vi "Micro-PL v10.4.1.vi"() -> ()   [LabVIEW 2010]
uses:
  drivers/Oxford ITC/ITCAPPS.LLB/ITCSetup.ctl
  drivers/Oxford ITC/ITCSUBS.LLB/ITCIO.ctl
  drivers/Oxford ITC/BUSGEN.LLB/OxfordAddress.ctl
  drivers/Oxford ITC/ITCSUBS.LLB/ITCVersion.ctl
  subvi/ESA-C/TypeDefs/ESA-C Live Controls v10.4.0.ctl
  subvi/ESA-C/TypeDefs/ESA-C Current Values.ctl
  subvi/ESA-C/TypeDefs/ESA-C Connection Settings.ctl
  subvi/ESA-C/TypeDefs/ESA-C Set Positions.ctl
  subvi/ITC503/TypeDefs/ITC503 Settings.ctl
  subvi/ITC503/TypeDefs/ITC503 Current Values.ctl
  subvi/iHR550/TypeDefs/iHR Current Values.ctl
  subvi/iHR550/TypeDefs/iHR Settings.ctl
  subvi/Mapping/TypeDefs/Mapping Spectra Params.ctl
  <vilib>/Utility/miscctls.llb/LVBoundsTypeDef.ctl
  <vilib>/Utility/miscctls.llb/LVPointTypeDef.ctl
  drivers/Horiba Spectrum One 3000V/Lib/CCD_command.llb/Comm Params.ctl
  subvi/Global Variables.vi
  <vilib>/Analysis/NI_AALBase.lvlib
panel:
  out "Spectrum Raw":dbl[][](array[numeric])
  out "Mapping State Storage":bool
  out "Mapping Reference":refnum<vi>
  out "Copy Drive Target":bool
  in  "CCD3500 Shutter":bool caption="Shutter:"
  out "Measurement Running":bool
  out "ITC503s Running":bool
  out "Drive Running":bool
  out "CCD3500V Running":bool
  out "iHR550 Running":bool
  in  "Exit":bool
  out "iHR550 Status":bool
  out "Drive Status":bool
  out "CCD3500V Status":bool
  out "ITC503 Status":bool
  in  "Register":enum32{"Devices", "Acquisition / Mapping"}(tab)
  out "iHR550 Timing":u32 caption="iHR550"
  out "Drive Timing":u32 caption="Drive"
  out "ITC Timing":u32 caption="ITC"
  out "CCD Timing":u32 caption="CCD"
  out "CCD3500 Temperature":dbl caption="Temp. (°C)" min=10.0 max=160.0 step=0.1 format="%.1f"
  in  "CCD3500V GPIB-Port":i32=5 caption="GPIB-Port" min=1 max=20 step=1 format="%#.0f"
  in  "CCD3500V Connect":bool
  in  "iHR550 Force Init":bool=TRUE
  in  "iHR550 Connect":bool
  in  "iHR550 ID":string(combo)="iHR550" caption="Monochromator ID"
  out "ITC503 Current Values":T1 {"ITC503 Gradient" format="%.2f"; "ITC503 Setpoint" min=-273.0 max=300000.0 step=0.0001 format="%.1f"; "ITC503 I" format="%_1f"; "ITC503 P" format="%_1f"; "ITC503 Temperature" min=0.0 max=1645.0 step=1e-05 format="%.2f"; "ITC503 Heater" min=0.0 max=100.0 step=0.01 scale=0.0..100.0}
  in  "ITC503 Settings":T2={"ITC503 Set Setpoint"=0.0, "ITC503 Set Auto Heater"=TRUE, "ITC503 Set Auto PID"=TRUE, "P"=0.0, "I"=0.0, "D"=0.0} {"D" min=0.0 max=100.0 step=0.1 format="%.1f"; "I" min=0.0 max=100.0 step=0.1 format="%.1f"; "P" min=0.0 max=100.0 step=0.1 format="%.1f"; "ITC503 Set Setpoint" min=-273.0 max=300000.0 step=0.1 format="%.1f"}
  in  "ITC503 Configure":bool
  in  "ITC503 Connect":bool
  in  "ITC503 Selector":u16(ring) caption="Select Device" items=["ITC503s"]
  out "Drive Current Values":T3 {"Position"."Drive Z Position" min=-273.0 max=300000.0 step=0.0001 format="%.1f"; "Position"."Drive Y Position" min=-273.0 max=300000.0 step=0.0001 format="%.1f"; "Position"."Drive X Position" min=-273.0 max=300000.0 step=0.0001 format="%.1f"; "Voltages"."Drive Z Voltage" min=-273.0 max=300000.0 step=0.0001 format="%.1f"; "Voltages"."Drive Y Voltage" min=-273.0 max=300000.0 step=0.0001 format="%.1f"; "Voltages"."Drive X Voltage" min=-273.0 max=300000.0 step=0.0001 format="%.1f"}
  in  "Drive Connection":T4={"Objective GPIB-Port"=4, "Stage GPIB-Port"=4, "Drive Selector"=0, "Drive Velocity (V/s)"=5.0} {"Drive Velocity (V/s)" min=10.0 max=160.0 step=0.1 format="%.1f"; "Drive Selector" items=["Obj.", "Stage"]; "Stage GPIB-Port" min=1 max=20 step=1 format="%#.0f"; "Objective GPIB-Port" min=1 max=20 step=1 format="%#.0f"}
  in  "Drive Connect":bool
  in  "Snapshot Folder":path=path "C:/Users/WET-KORR/Desktop/Screenshots"
  in  "Camera Name":string="HD USB Camera"
  in  "Spectrum Noise":i64 caption="Noise Level"
  in  "Wavelength Switch":bool
  out "Spectrum":cluster{dbl[], dbl[]}[](graph)
  in  "Spectrum Load":bool
  in  "Spectrum Save":bool
  in  "CCD3000 Current Rep.":string="0/0"
  in  "Spectrum Maximize":bool
  in  "Video Show":bool
  in  "Drive GoTo":bool caption="Objective Move Abs."
  in  "Drive New Positions":T5 {"Drive X Set" min=10.0 max=160.0 step=0.1 format="%.1f"; "Drive Z Set" min=10.0 max=160.0 step=0.1 format="%.1f"; "Drive Y Set" min=10.0 max=160.0 step=0.1 format="%.1f"}
  in  "Spectrum Autosave":bool caption="iHR550 Force Init"
  in  "CCD3500 Preview":bool
  in  "CCD3500 Acquire":bool
  in  "Spectra Settings":T6={"Integration Time"=1.0, "Repetitions"=1, "Mapping Spectra"=TRUE} caption="Mapping Spectra Settings" {"Repetitions" min=1 max=100 step=1; "Integration Time" min=0.1 max=6000.0 step=0.1 format="%.1f"}
  in  "Mapping Start":bool
  in  "iHR550 Configure":bool
  in  "iHR Settings":T7={"iHR550 Set Exit Mirror"=2, "iHR550 Set Side Exit"=0.0, "iHR550 Set Front Entrance"=0.0, "iHR550 Set Wavelength"=897.9988, "iHR550 Set Grating"=0, "iHR550 Set Grating Switch"=FALSE, "iHR550 Set Wavelength Switch"=FALSE, "iHR550 Set Mirror Switch"=FALSE, "iHR550 Set Slits Switch"=FALSE} {"iHR550 Set Grating" items=["1800"=1, "600"=2, "150"=3]; "iHR550 Set Wavelength" min=0.0 max=1500.0 step=1.0; "iHR550 Set Side Exit" min=0.0 max=2000.0 step=1.0; "iHR550 Set Exit Mirror" items=["Front"=2, "Side"=3]}
  out "iHR Current Values":T8={"iHR 550 Front Entrance"=0.0, "iHR550 Side Exit"=0.0, "iHR550 Wavelength"=897.9988, "iHR550 Exit Mirror"=2, "iHR550 Grating"="1", "Grating Index"=1} {"iHR550 Exit Mirror" items=["EntranceMirror", "ExitMirror", "Front", "Side"]}
  out "Drive Live Current Values":T3 {"Position"."Drive Z Position" min=-273.0 max=300000.0 step=0.0001 format="%.1f"; "Position"."Drive Y Position" min=-273.0 max=300000.0 step=0.0001 format="%.1f"; "Position"."Drive X Position" min=-273.0 max=300000.0 step=0.0001 format="%.1f"; "Voltages"."Drive Z Voltage" min=-273.0 max=300000.0 step=0.0001 format="%.1f"; "Voltages"."Drive Y Voltage" min=-273.0 max=300000.0 step=0.0001 format="%.1f"; "Voltages"."Drive X Voltage" min=-273.0 max=300000.0 step=0.0001 format="%.1f"}
  in  "Drive Live Controls":T9={"Move Step"=1.0, "Move Home"=FALSE, "Move Down"=FALSE, "Move Up"=FALSE, "Move Left"=FALSE, "Move Right"=FALSE, "Move Out"=FALSE, "Move In"=FALSE} {"Move Step" min=0.0 max=30.0 step=0.1 format="%.1f"}
  out "ITC503 Temp Storage":dbl
  out "Runtime":u32
  out "ITC Gradient Time":i64
  out "Read ITC":bool
  out "Read CCD3500":bool
  out "Read iHR550":bool
  out "Read Drive":bool
  out "Spectrum Properties":cluster{"Position":T10, "Plot Area Size":T10}={"Position"={"Width"=36, "Height"=367}, "Plot Area Size"={"Width"=496, "Height"=264}}
  in  "Auto Folder":path caption="Ausgewählter Pfad"
  out "Int. Time Temp":dbl
  out "Wavelengths (nm)":dbl[](array[numeric])
  in  "CCD3500V Connection":T11={"Comm Interface"=1, "BUS"=0, "Address"=5, "Com Port"=0}
  out "Video Running":bool
  out "iHR550 RefNum":refnum<k7> caption="Mono RefNum out"
  out "ITC Setup":T12={"Description"="", "IO Info"={"Address"={"Com Port"=1, "ISOBUS Address"=1, "GPIB Address"=24, "Communication"=enum."ISOBUS"}, "Version"=enum."ITC503", "Ch 1 dec places"=1, "Ch 2 dec places"=1, "Ch 3 dec places"=1, "Ch1 Name"="", "Ch2 Name"="", "Ch3 Name"=""}}
  # "Correlation Setup"
  # "Active"
  # "Active"
  # "ITC"
  # "iHR"
  # "Drive"
  # "CCD"
  # "Status"
  # "CCD"
  # "ITC"
  # "iHR"
  # "Drive"
  # "Timing"
  # "CCD"
  # "Monochromator"
  # "Cryostat"
  # "Drives"
  # "Video"
  # "Drive Control"
  # "Spectrum"
  # "CCD"
  # "Mapping"
  # "Launch the Spectral Mapping VI and Raman Tool Set 2.0 in a new window."
  # "Monochromator"
  # "XY"
  # "Z"
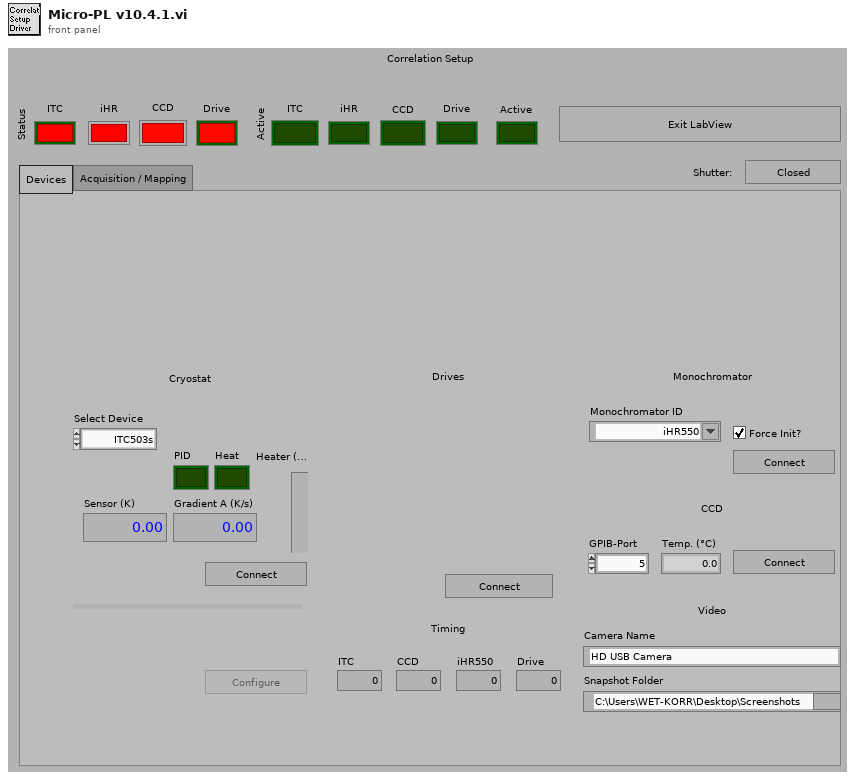
[diagram p1: front panel]
types:
  T1 = typedef "ITC503 Current Values.ctl" = cluster{"ITC503 Heater":dbl, "ITC503 Temperature":dbl, "ITC503 P":dbl, "ITC503 I":dbl, "ITC503 D":dbl, "ITC503 Setpoint":dbl, "ITC503 Gradient":dbl, "ITC503 Heater Auto":bool, "ITC503 PID Auto":bool}
  T2 = typedef "ITC503 Settings.ctl" = cluster{"ITC503 Set Setpoint":dbl, "ITC503 Set Auto Heater":bool, "ITC503 Set Auto PID":bool, "P":dbl, "I":dbl, "D":dbl}
  T3 = typedef "ESA-C Current Values.ctl" = cluster{"Voltages":cluster{"Drive X Voltage":dbl, "Drive Y Voltage":dbl, "Drive Z Voltage":dbl}, "Position":cluster{"Drive X Position":dbl, "Drive Y Position":dbl, "Drive Z Position":dbl}}
  T4 = typedef "ESA-C Connection Settings.ctl" = cluster{"Objective GPIB-Port":i32, "Stage GPIB-Port":i32, "Drive Selector":u16, "Drive Velocity (V/s)":dbl}
  T5 = typedef "ESA-C Set Positions.ctl" = cluster{"Drive X Set":dbl, "Drive Y Set":dbl, "Drive Z Set":dbl}
  T6 = typedef "Mapping Spectra Params.ctl" = cluster{"Integration Time":dbl, "Repetitions":u16, "Mapping Spectra":bool}
  T7 = typedef "iHR Settings.ctl" = cluster{"iHR550 Set Exit Mirror":u16, "iHR550 Set Side Exit":dbl, "iHR550 Set Front Entrance":dbl, "iHR550 Set Wavelength":dbl, "iHR550 Set Grating":u16, "iHR550 Set Grating Switch":bool, "iHR550 Set Wavelength Switch":bool, "iHR550 Set Mirror Switch":bool, "iHR550 Set Slits Switch":bool}
  T8 = typedef "iHR Current Values.ctl" = cluster{"iHR 550 Front Entrance":dbl, "iHR550 Side Exit":dbl, "iHR550 Wavelength":dbl, "iHR550 Exit Mirror":i32, "iHR550 Grating":string, "Grating Index":i32}
  T9 = typedef "ESA-C Live Controls v10.4.0.ctl" = cluster{"Move Step":dbl, "Move Home":bool, "Move Down":bool, "Move Up":bool, "Move Left":bool, "Move Right":bool, "Move Out":bool, "Move In":bool}
  T10 = typedef "LVBoundsTypeDef.ctl" = cluster{"Width":u32, "Height":u32}
  T11 = cluster{"Comm Interface":u16, "BUS":i16, "Address":i16, "Com Port":i32}
  T12 = typedef "ITCSetup.ctl" = cluster{"Description":string, "IO Info":T13}
  T13 = typedef "ITCIO.ctl" = cluster{"Address":T14, "Version":T15, "Ch 1 dec places":i16, "Ch 2 dec places":i16, "Ch 3 dec places":i16, "Ch1 Name":string, "Ch2 Name":string, "Ch3 Name":string}
  T14 = typedef "OxfordAddress.ctl" = cluster{"Com Port":i32, "ISOBUS Address":i32, "GPIB Address":i16, "Communication":enum16{"RS232", "ISOBUS", "GPIB", "Gateway"}}
  T15 = typedef "ITCVersion.ctl" = enum16{"ITC502", "ITC503", "ITC601"}
  T16 = typedef "LVPointTypeDef.ctl" = cluster{"Horizontal":i16, "Vertical":i16}
  T17 = enum8{"Enabled", "Disabled", "Disabled and Grayed Out"}
  T18 = typedef "Comm Params.ctl" = cluster{"Comm Interface":u16, "BUS":i16, "Address":i16, "Com Port":i32}
  T19 = enum16{"CCD Temperature Z345", "CCD Temperature Z308", "CCD Gain"}
  T20 = cluster{"CCD3000 Connection":T18, "Drive Connection Settings":T4, "ITC503 Current Values":T1, "Wavelengths (nm)":dbl[], "Drive Current Values":T3, "iHR Current Values":T8, "Spectra Settings":T6, "CCD3500 Temperature":dbl, "Simulate Drive 2":bool, "Simulate Spectra 2":bool}
  T21 = cluster{"Drive X Position":dbl, "Drive Y Position":dbl, "Drive Z Position":dbl}
  T22 = cluster{"Intensities":dbl[], "Wavelengths":dbl[]}[]
  T23 = typedef "LVPositionTypeDef.ctl" = cluster{"Left":i32, "Top":i32}
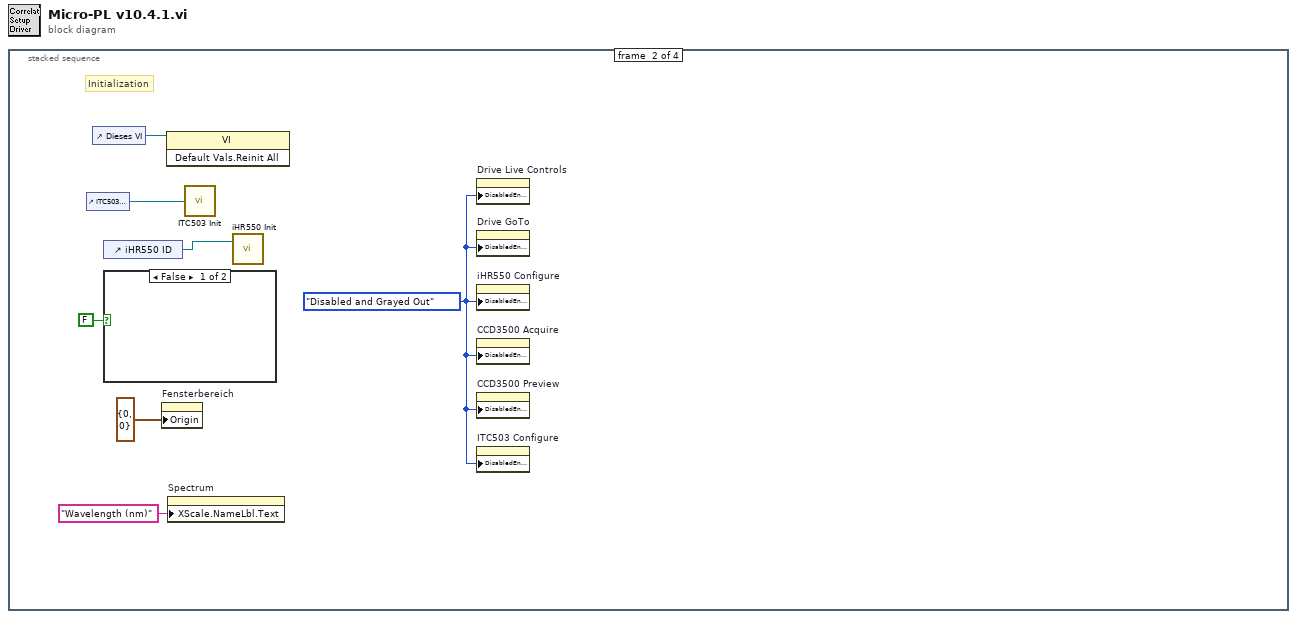
[diagram p0: block diagram]
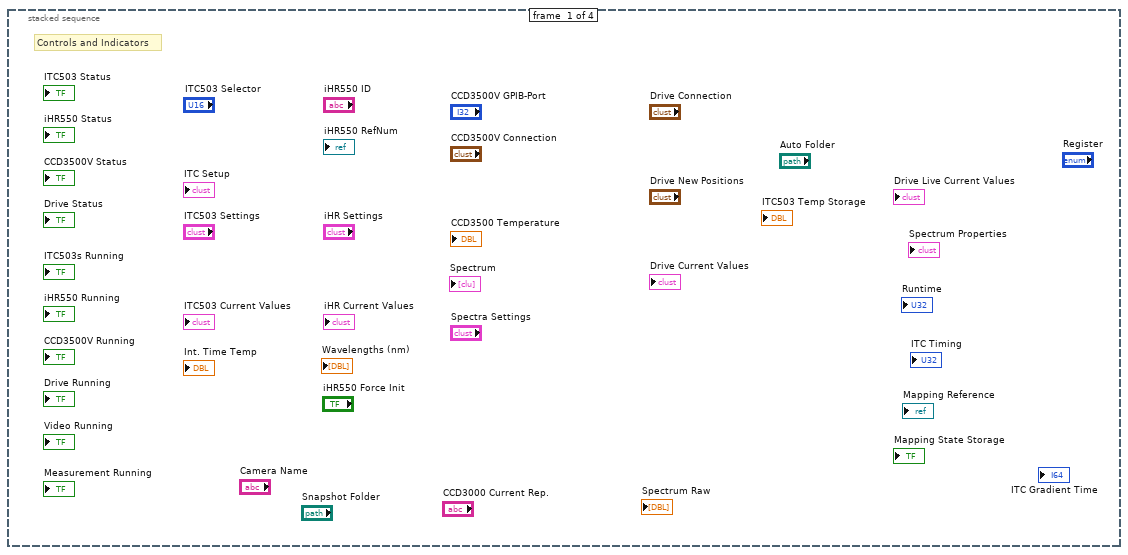
[diagram p2: hidden frame]
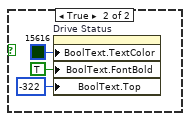
[diagram p3: hidden frame]
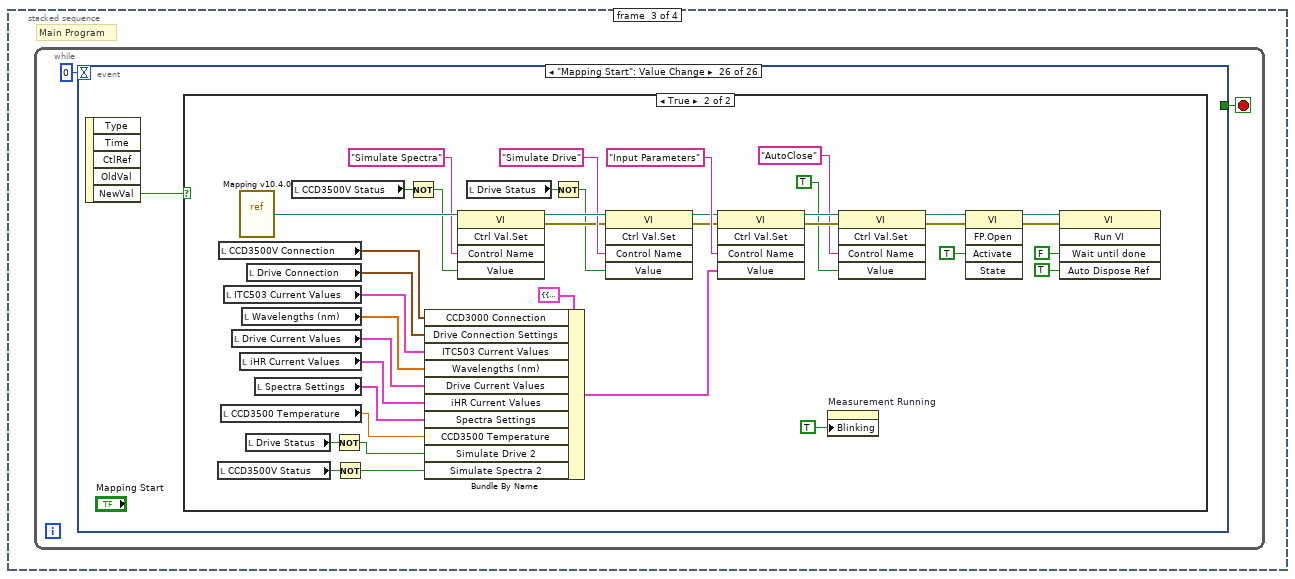
[diagram p4: hidden frame]
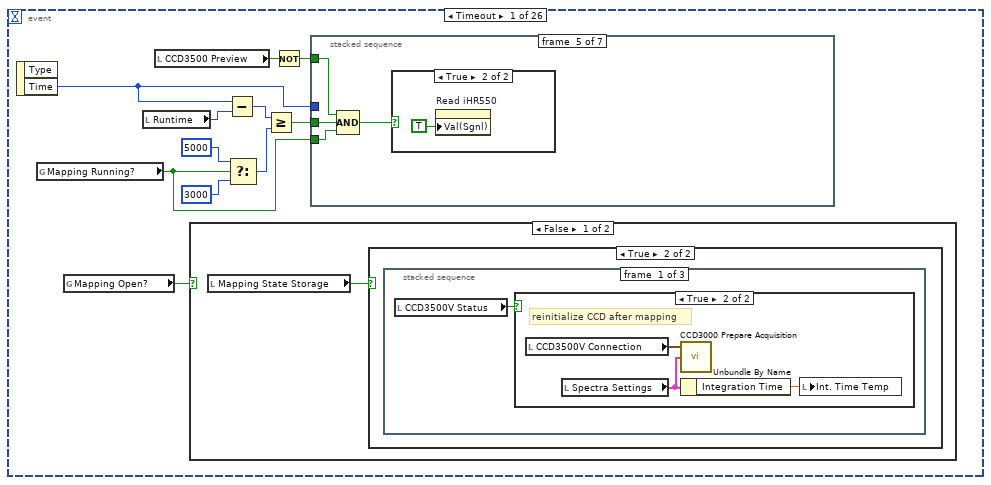
[diagram p5: hidden frame]
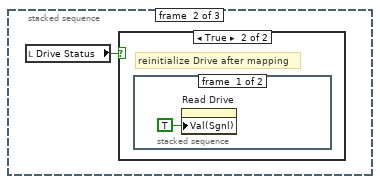
[diagram p8: hidden frame]
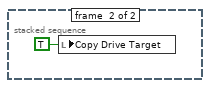
[diagram p10: hidden frame]
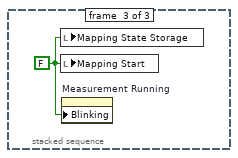
[diagram p11: hidden frame]
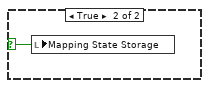
[diagram p12: hidden frame]
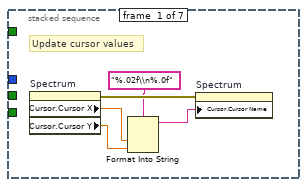
[diagram p13: hidden frame]
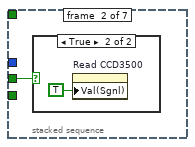
[diagram p14: hidden frame]
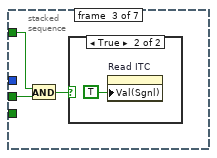
[diagram p16: hidden frame]
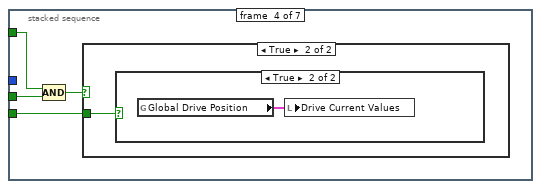
[diagram p18: hidden frame]
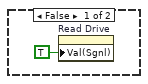
[diagram p20: hidden frame]
diagram:
  n1 = stacked-sequence {
    frame #0 {
      # "Controls and Indicators"
    }
    frame #1 {
      w2 = T17."Disabled and Grayed Out" ("Deaktiviert")
      # "Initialization"
      n2 = control-ref of="ITC503 Selector"() -> (w7:refnum<vi>)
      n3 = control-ref of="Dieses VI"() -> (w6:refnum<vi>)
      n4 = control-ref of="iHR550 ID"() -> (w5:refnum<vi>)
      n5 = case shown="False" FALSE {
        frame False {
        }
        frame True {
          n6 = property on="Drive Status" class="Bool (strict)"("BoolText.TextColor"=u32 15616, "BoolText.FontBold"=TRUE ("Boolescher Text.Schriftart:Fett"), "BoolText.Top"=-322 ("Boolescher Text.Position:Oben")) -> ()  [unwired: 2 in, 2 out]
        }
      }
      n7 = property on="Fensterbereich" class="Pane"("Origin"=T16 {"Horizontal"=0, "Vertical"=0}) -> ()  [unwired: 2 in, 2 out]
      n8 = invoke class="VI" method="Default Vals.Reinit All"(reference=w6) -> ()  [unwired: 2 in, 3 out]
      n9 = property on="Spectrum" class="XYGraph (strict)"("XScale.NameLbl.Text"="Wavelength (nm)" ("X Scale.Name Label.Text")) -> ()  [unwired: 2 in, 2 out]
      n10 = call "ITC503 Init.vi"("ITC Selector"=w7) -> ()  [unwired: 1 in]
      n11 = call "iHR550 Init.vi"("Mono ID"=w5) -> ()  [unwired: 2 in]
      n12 = property on="Drive Live Controls" class="Clust (strict)"("DisabledEnum"=w2) -> ()  [unwired: 2 in, 2 out]
      n13 = property on="Drive GoTo" class="Bool (strict)"("DisabledEnum"=w2) -> ()  [unwired: 2 in, 2 out]
      n14 = property on="iHR550 Configure" class="Bool (strict)"("DisabledEnum"=w2) -> ()  [unwired: 2 in, 2 out]
      n15 = property on="CCD3500 Acquire" class="Bool (strict)"("DisabledEnum"=w2) -> ()  [unwired: 2 in, 2 out]
      n16 = property on="CCD3500 Preview" class="Bool (strict)"("DisabledEnum"=w2) -> ()  [unwired: 2 in, 2 out]
      n17 = property on="ITC503 Configure" class="Bool (strict)"("DisabledEnum"=w2) -> ()  [unwired: 2 in, 2 out]
    }
    frame #2 {
      # "Main Program"
      n18 = while "Main-Program" {
        stop <- w12 stop-if-true
        n19 = event shown="[25] \"Mapping Start\": Value Change" {
          selector: _ -> [_ _ _ _ _ _ _ _ _ _ _ _ _ _ _ _ _ _ _ _ _ _ _ _ _ _]
          dyn-events: _ -> [_ _ _ _ _ _ _ _ _ _ _ _ _ _ _ _ _ _ _ _ _ _ _ _ _ _]
          timeout: 0 -> [_ _ _ _ _ _ _ _ _ _ _ _ _ _ _ _ _ _ _ _ _ _ _ _ _ _]
          tunnel: [_ w62 _ _ _ _ _ _ _ _ _ _ _ _ _ _ _ _ _ _ _ _ _ _ _ _] -> w12
          event Timeout {
            n20 = event-data() -> ("Time"=w19:u32)  [unwired: 1 in, 1 out]
            n21 = global read "Global Variables.vi" "Mapping Running?"() -> (w14:bool)
            n22 = global read "Global Variables.vi" "Mapping Open?"() -> (w13:bool)
            n23 = local read "Runtime"() -> (w18:u32)
            n24 = local read "CCD3500 Preview"() -> (w21:bool)
            n25 = case shown="False" w13 {
              selector: w13 -> [_ w33]
              frame False {
                n26 = local read "Mapping State Storage"() -> (w24:bool)
                n27 = case shown="True" w24 {
                  frame False {
                  }
                  frame True {
                    n28 = stacked-sequence {
                      frame #0 {
                        n29 = local read "CCD3500V Status"() -> (w25:bool)
                        n30 = case shown="True" w25 {
                          frame False {
                          }
                          frame True {
                            # "reinitialize CCD after mapping"
                            n31 = local read "CCD3500V Connection"() -> (w26:T11)
                            n32 = local read "Spectra Settings"() -> (w28:T6)
                            n33 = call "CCD3000 Prepare Acquisition.vi"("Mapping Spectra Settings"=w28, "Comm Params"=w26) -> ()  [unwired: 4 in]
                            n34 = Unbundle By Name(w28) -> ("Integration Time"=w27:dbl)
                            n35 = local write "Int. Time Temp"(w27) -> ()
                          }
                        }
                      }
                      frame #1 {
                        n36 = local read "Drive Status"() -> (w29:bool)
                        n37 = case shown="True" w29 {
                          frame False {
                          }
                          frame True {
                            # "reinitialize Drive after mapping"
                            n38 = stacked-sequence {
                              frame #0 {
                                n39 = property on="Read Drive" class="Bool (strict)"("Val(Sgnl)"=TRUE ("Value (Signaling)")) -> ()  [unwired: 2 in, 2 out]
                              }
                              frame #1 {
                                n40 = local write "Copy Drive Target"(TRUE ("Copy Drive Target")) -> ()
                              }
                            }
                          }
                        }
                      }
                      frame #2 {
                        w32 = FALSE ("Mapping Start")
                        n41 = local write "Mapping State Storage"(w32) -> ()
                        n42 = local write "Mapping Start"(w32) -> ()
                        n43 = property on="Measurement Running" class="Bool (strict)"("Blinking"=w32) -> ()  [unwired: 2 in, 2 out]
                      }
                    }
                  }
                }
              }
              frame True {
                n44 = local write "Mapping State Storage"(w33) -> ()
              }
            }
            n45 = Subtract(x=w19, y=w18) -> (x-y=w22:u32)
            n46 = Select(t=u32 5000 ("y"), s=w14, f=u32 3000 ("y")) -> (s? t:f=w15:u32)
            n47 = Greater Or Equal?(x=w22, y=w15) -> (x >= y?=w23:bool)
            n48 = Not(x=w21) -> (.not. x?=w20:bool)
            n49 = stacked-sequence {
              tunnel: w23 -> [_ w39 w43 w48 w55 _ w59]
              tunnel: w19 -> [_ _ _ _ _ _ w60]
              tunnel: w20 -> [_ _ w42 w47 w54 w57 _]
              tunnel: w14 -> [_ _ _ w45 w52 _ _]
              frame #0 {
                # "Update cursor values"
                n50 = property on="Spectrum" class="XYGraph (strict)"() -> (error out=w38:errorcluster, "Cursor.Cursor X"=w37:dbl, "Cursor.Cursor Y"=w36:dbl)  [unwired: 2 in, 1 out]
                n51 = Format Into String(format string="%.02f\\n%.0f", w37, w36) -> (resulting string=w34:string)  [unwired: 2 in, 1 out]
                n52 = property on="Spectrum" class="XYGraph (strict)"(error in=w38, "Cursor.Cursor Name"=w34) -> ()  [unwired: 1 in, 2 out]
              }
              frame #1 {
                n53 = case shown="True" w39 {
                  frame False {
                  }
                  frame True {
                    n54 = property on="Read CCD3500" class="Bool (strict)"("Val(Sgnl)"=TRUE ("Value (Signaling)")) -> ()  [unwired: 2 in, 2 out]
                  }
                }
              }
              frame #2 {
                n55 = And(x=w42, y=w43) -> (x .and. y?=w41:bool)
                n56 = case shown="True" w41 {
                  frame False {
                  }
                  frame True {
                    n57 = property on="Read ITC" class="Bool (strict)"("Val(Sgnl)"=TRUE ("Value (Signaling)")) -> ()  [unwired: 2 in, 2 out]
                  }
                }
              }
              frame #3 {
                n58 = Compound Arithmetic op=AND(w47, w48) -> (w46:bool)
                n59 = case shown="True" w46 {
                  tunnel: w45 -> [_ w49]
                  frame False {
                  }
                  frame True {
                    n60 = case shown="True" w49 {
                      frame False {
                        n61 = property on="Read Drive" class="Bool (strict)"("Val(Sgnl)"=TRUE ("Value (Signaling)")) -> ()  [unwired: 2 in, 2 out]
                      }
                      frame True {
                        n62 = global read "Global Variables.vi" "Global Drive Position"() -> (w51:T3)
                        n63 = local write "Drive Current Values"(w51) -> ()
                      }
                    }
                  }
                }
              }
              frame #4 {
                n64 = Compound Arithmetic op=AND(w54, w55, w52) -> (w53:bool)
                n65 = case shown="True" w53 {
                  frame False {
                  }
                  frame True {
                    n66 = property on="Read iHR550" class="Bool (strict)"("Val(Sgnl)"=TRUE ("Value (Signaling)")) -> ()  [unwired: 2 in, 2 out]
                  }
                }
              }
              frame #5 {
                n67 = case shown="False" w57 {
                  frame False {
                    n68 = property on="CCD3500 Acquire" class="Bool (strict)"("Val(Sgnl)"=TRUE ("Wert (signalisierend)")) -> ()  [unwired: 2 in, 2 out]
                  }
                  frame True {
                  }
                }
              }
              frame #6 {
                # "Set runtime counter"
                n69 = case shown="True" w59 {
                  tunnel: w60 -> [_ w61]
                  frame False {
                  }
                  frame True {
                    n70 = local write "Runtime"(w61) -> ()
                  }
                }
              }
            }
          }
          event "Exit": Value Change {
            n71 = event-data() -> ("NewVal"=w62:bool)  [unwired: 1 in, 4 out]
          }
          event "ITC503 Connect": Value Change {
            n72 = event-data() -> ("NewVal"=w63:bool)  [unwired: 1 in, 4 out]
            n73 = stacked-sequence {
              tunnel: w63 -> [_ w65 _]
              frame #0 {
                n74 = property on="ITC503s Running" class="Bool (strict)"("Blinking"=TRUE ("Blinkend")) -> ()  [unwired: 2 in, 2 out]
              }
              frame #1 {
                n75 = case shown="True" w65 {
                  selector: w65 -> [w70 _]
                  tunnel: [w70 w77] -> w67
                  frame False {
                    # "disconnect"
                    n76 = control-ref of="ITC503s Running"() -> (w71:refnum<vi>)
                    n77 = property class="Bool (strict)"(reference=w71, "Blinking"=w70, "Value"=w70) -> ()  [unwired: 1 in, 2 out]
                  }
                  frame True {
                    # "connect"
                    n78 = local read "ITC503 Selector"() -> (w78:u16)
                    n79 = call "ITC503 Connect.vi"("ITC Selector"=w78) -> ("ITC Setup"=w76:T12, "Connected"=w77:bool)
                    n80 = local write "ITC Setup"(w76) -> ()
                    n81 = call "ITC503 Get Values.vi"("ITC Setup"=w76) -> ("ITC503 Current Values"=w75:T1)  [unwired: 1 in, 1 out]
                    n82 = Unbundle By Name(w75) -> ("ITC503 Setpoint"=w72:dbl)
                    n83 = Bundle By Name(cluster=T2 {"ITC503 Set Setpoint"=0.0, "ITC503 Set Auto Heater"=TRUE, "ITC503 Set Auto PID"=TRUE, "P"=0.0, "I"=0.0, "D"=0.0} ("ITC503 Settings"), "ITC503 Set Setpoint"=w72) -> (w73:T2)
                    n84 = local write "ITC503 Settings"(w73) -> ()
                  }
                }
                n85 = case shown="False" w67 {
                  tunnel: [T17."Disabled and Grayed Out" ("Deaktiviert") T17."Enabled" ("Deaktiviert")] -> w66
                  frame False {
                  }
                  frame True {
                  }
                }
                n86 = local write "ITC503 Status"(w67) -> ()
                n87 = local write "ITC503 Connect"(w67) -> ()
                n88 = property on="ITC503 Configure" class="Bool (strict)"("DisabledEnum"=w66) -> ()  [unwired: 2 in, 2 out]
              }
              frame #2 {
                n89 = property on="ITC503s Running" class="Bool (strict)"("Blinking"=FALSE ("Blinkend")) -> ()  [unwired: 2 in, 2 out]
                n90 = property on="Read ITC" class="Bool (strict)"("Val(Sgnl)"=TRUE ("Wert (signalisierend)")) -> ()  [unwired: 2 in, 2 out]
              }
            }
          }
          event "Read ITC": Value Change {
            n91 = event-data() -> ("Time"=w82:u32, "NewVal"=w86:bool)  [unwired: 1 in, 3 out]
            n92 = local read "ITC503 Status"() -> (w85:bool)
            n93 = control-ref of="ITC503s Running"() -> (w83:refnum<vi>)
            n94 = And(x=w85, y=w86) -> (x .and. y?=w84:bool)
            n95 = case shown="True" w84 {
              tunnel: w83 -> [w88 w92]
              tunnel: w82 -> [_ w91]
              tunnel: [u32 0 w90] -> w81
              frame False {
                n96 = property class="Bool (strict)"(reference=w88, "BoolText.Text"="" ("Boolescher Text.Text")) -> ()  [unwired: 1 in, 2 out]
              }
              frame True {
                n97 = stacked-sequence {
                  seq-local: [_ w98 _ _] -> [_ _ w114 _]
                  seq-local: [w93 _ _ _] -> [_ _ _ w120]
                  tunnel: w92 -> [_ _ w107 _]
                  tunnel: w91 -> [_ w99 _ _]
                  tunnel: [_ _ _ w121] -> w90
                  frame #0 {
                    n98 = Tick Count (ms)() -> (millisecond timer value=w93:u32)
                  }
                  frame #1 {
                    n99 = local read "ITC Setup"() -> (w105:T12)
                    n100 = local read "ITC Gradient Time"() -> (w103:i64)
                    n101 = call "ITC503 Get Values.vi"("ITC Setup"=w105) -> ("ITC503 Current Values"=w98:T1)  [unwired: 1 in, 1 out]
                    n102 = local read "ITC503 Temp Storage"() -> (w97:dbl)
                    n103 = Unbundle By Name(w98) -> ("ITC503 Temperature"=w95:dbl)
                    n104 = Subtract(x=w99, y=w103) -> (x-y=w102:i64)
                    n105 = Divide(x=w102, y=i64 1000) -> (x/y=w100:dbl)
                    n106 = Subtract(x=w95, y=w97) -> (x-y=w96:dbl)
                    n107 = Divide(x=w96, y=w100) -> (x/y=w104:dbl)
                    n108 = Bundle By Name(cluster=w98, "ITC503 Gradient"=w104) -> (w94:T1)
                    n109 = local write "ITC503 Current Values"(w94) -> ()
                    n110 = global write "Global Variables.vi" "Global ITC Values"(w94) -> ()
                  }
                  frame #2 {
                    n111 = Unbundle By Name(w114) -> ("ITC503 Temperature"=w106:dbl, "ITC503 Setpoint"=w115:dbl)
                    n112 = Subtract(x=w106, y=w115) -> (x-y=w116:dbl)
                    n113 = Number To Fractional String(number=w106, precision (6)=i16 2 ("Genauigkeit (6)")) -> (F-format string=w110:string)  [unwired: 2 in]
                    n114 = Absolute Value(x=w116) -> (abs(x)=w117:dbl)
                    n115 = String Subset(string=w110, length (rest)=5 ("Länge (Rest)")) -> (substring=w108:string)  [unwired: 1 in]
                    n116 = Greater?(x=w117, y=2.0) -> (0:w113:bool)
                    n117 = Not(x=w113) -> (.not. x?=w112:bool)
                    n118 = property class="Bool (strict)"(reference=w107, "Blinking"=w113, "Value"=w112, "BoolText.Text"=w108) -> ()  [unwired: 1 in, 2 out]
                    n119 = local write "ITC503 Temp Storage"(w106) -> ()
                  }
                  frame #3 {
                    n120 = Tick Count (ms)() -> (millisecond timer value=w119:u32)
                    n121 = local write "ITC Gradient Time"(w119) -> ()
                    n122 = Subtract(x=w119, y=w120) -> (x-y=w121:u32)
                  }
                }
              }
            }
            n123 = local write "ITC Timing"(w81) -> ()
          }
          event "iHR550 Connect": Value Change {
            n124 = event-data() -> ("NewVal"=w122:bool)  [unwired: 1 in, 4 out]
            n125 = stacked-sequence {
              tunnel: w122 -> [_ w125 _]
              frame #0 {
                n126 = property on="iHR550 Running" class="Bool (strict)"("Blinking"=TRUE ("Blinkend")) -> ()  [unwired: 2 in, 2 out]
              }
              frame #1 {
                n127 = case shown="True" w125 {
                  selector: w125 -> [w129 _]
                  tunnel: [w129 w142] -> w124
                  frame False {
                    # "disconnect"
                  }
                  frame True {
                    # "connect"
                    n128 = local read "iHR550 Force Init"() -> (w140:bool)
                    n129 = control-ref of="iHR550 Set Grating"() -> (w141:refnum<vi>)
                    n130 = local read "iHR550 ID"() -> (w143:string)
                    n131 = call "iHR550 Connect.vi"("Force\nInitialization"=w140, "Grating Selector"=w141, "Mono ID"=w143) -> ("Initialized"=w142:bool, "iHR550 RefNum"=w139:refnum<k7>)  [unwired: 2 in, 4 out]
                    n132 = local write "iHR550 RefNum"(w139) -> ()
                    n133 = call "iHR550 Read Values.vi"("JYMONOLib.IJYMonoReqd"=w139) -> ("iHR Current Values"=w131:T8)  [unwired: 1 in]
                    n134 = local write "iHR Current Values"(w131) -> ()
                    n135 = Unbundle By Name(w131) -> ("iHR 550 Front Entrance"=w137:dbl, "iHR550 Side Exit"=w136:dbl, "iHR550 Wavelength"=w135:dbl, "iHR550 Exit Mirror"=w134:i32, "Grating Index"=w132:i32)
                    n136 = call "iHR550 Convert Axis.vi"("iHR Current Values"=w131) -> ("Wavelengths (nm)"=w130:dbl[])
                    n137 = local write "Wavelengths (nm)"(w130) -> ()
                    n138 = Bundle By Name(cluster=T7 {"iHR550 Set Exit Mirror"=0, "iHR550 Set Side Exit"=0.0, "iHR550 Set Front Entrance"=0.0, "iHR550 Set Wavelength"=0.0, "iHR550 Set Grating"=0, "iHR550 Set Grating Switch"=FALSE, "iHR550 Set Wavelength Switch"=FALSE, "iHR550 Set Mirror Switch"=FALSE, "iHR550 Set Slits Switch"=FALSE} ("iHR Settings"), "iHR550 Set Front Entrance"=w137, "iHR550 Set Side Exit"=w136, "iHR550 Set Wavelength"=w135, "iHR550 Set Exit Mirror"=w134, "iHR550 Set Grating"=w132) -> (w133:T7)
                    n139 = local write "iHR Settings"(w133) -> ()
                  }
                }
                n140 = local write "iHR550 Status"(w124) -> ()
                n141 = local write "iHR550 Connect"(w124) -> ()
                n142 = case shown="False" w124 {
                  tunnel: [T17."Disabled and Grayed Out" ("Deaktiviert") T17."Enabled" ("Deaktiviert")] -> w126
                  frame False {
                  }
                  frame True {
                  }
                }
                n143 = property on="iHR550 Configure" class="Bool (strict)"("DisabledEnum"=w126) -> ()  [unwired: 2 in, 2 out]
              }
              frame #2 {
                n144 = local write "iHR550 Force Init"(FALSE ("iHR550 Force Init")) -> ()
                n145 = property on="iHR550 Running" class="Bool (strict)"("Blinking"=FALSE ("Blinkend")) -> ()  [unwired: 2 in, 2 out]
                n146 = property on="Read iHR550" class="Bool (strict)"("Val(Sgnl)"=TRUE ("Wert (signalisierend)")) -> ()  [unwired: 2 in, 2 out]
              }
            }
          }
          event "Read iHR550": Value Change {
            n147 = event-data() -> ("NewVal"=w150:bool)  [unwired: 1 in, 4 out]
            n148 = local read "iHR550 Status"() -> (w149:bool)
            n149 = And(x=w149, y=w150) -> (x .and. y?=w148:bool)
            n150 = case shown="True" w148 {
              tunnel: [u32 0 w152] -> w147
              frame False {
              }
              frame True {
                n151 = stacked-sequence {
                  seq-local: [w153 _ _] -> [_ _ w156]
                  tunnel: [_ _ w157] -> w152
                  frame #0 {
                    n152 = Tick Count (ms)() -> (millisecond timer value=w153:u32)
                  }
                  frame #1 {
                    n153 = local read "iHR550 RefNum"() -> (w155:refnum<k7>)
                    n154 = call "iHR550 Read Values.vi"("JYMONOLib.IJYMonoReqd"=w155) -> ("iHR Current Values"=w154:T8)  [unwired: 1 in]
                    n155 = local write "iHR Current Values"(w154) -> ()
                    n156 = global write "Global Variables.vi" "Global iHR Values"(w154) -> ()
                  }
                  frame #2 {
                    n157 = Tick Count (ms)() -> (millisecond timer value=w158:u32)
                    n158 = Subtract(x=w158, y=w156) -> (x-y=w157:u32)
                  }
                }
              }
            }
            "iHR550 Timing" <- w147
          }
          event "CCD3500V Connect": Value Change {
            n159 = event-data() -> ("NewVal"=w159:bool)  [unwired: 1 in, 4 out]
            n160 = stacked-sequence {
              tunnel: w159 -> [_ w161 _]
              frame #0 {
                n161 = property on="CCD3500V Running" class="Bool (strict)"("Blinking"=TRUE ("Blinkend")) -> ()  [unwired: 2 in, 2 out]
              }
              frame #1 {
                n162 = case shown="True" w161 {
                  selector: w161 -> [w167 _]
                  tunnel: [w167 w168] -> w163
                  frame False {
                    # "disconnect"
                    n163 = local read "CCD3500V Connection"() -> (w166:T11)
                    n164 = call "CCDSTOP.VI"("Comm Params"=w166) -> ()  [unwired: 1 out]
                  }
                  frame True {
                    # "connect"
                    n165 = stacked-sequence {
                      seq-local: [_ w172 _] -> [_ _ w174]
                      tunnel: [_ w173 _] -> w168
                      frame #0 {
                        n166 = local read "CCD3500V GPIB-Port"() -> (w170:i32)
                        n167 = Bundle By Name(cluster=T18 {"Comm Interface"=1, "BUS"=0, "Address"=5, "Com Port"=1} ("Comm Params"), "Address"=w170) -> (w171:T18)
                        n168 = local write "CCD3500V Connection"(w171) -> ()
                      }
                      frame #1 {
                        n169 = local read "CCD3500V Connection"() -> (w172:T11)
                        n170 = call "CCD3000 Initialize.vi"("Comm Params"=w172) -> ("Success"=w173:bool)  [unwired: 9 in, 1 out]
                      }
                      frame #2 {
                        n171 = local read "Spectra Settings"() -> (w175:T6)
                        n172 = Unbundle By Name(w175) -> ("Integration Time"=w176:dbl)
                        n173 = local write "Int. Time Temp"(w176) -> ()
                        n174 = call "CCD3000 Prepare Acquisition.vi"("Mapping Spectra Settings"=w175, "Comm Params"=w174) -> ()  [unwired: 4 in]
                      }
                    }
                  }
                }
                n175 = local write "CCD3500V Connect"(w163) -> ()
                n176 = local write "CCD3500V Status"(w163) -> ()
                n177 = case shown="False" w163 {
                  tunnel: [T17."Disabled and Grayed Out" ("Deaktiviert") T17."Enabled" ("Deaktiviert")] -> w162
                  frame False {
                  }
                  frame True {
                  }
                }
                n178 = property on="CCD3500V Status" class="Bool (strict)"("BoolText.Visible"=w163) -> ()  [unwired: 2 in, 2 out]
                n179 = property on="CCD3500 Acquire" class="Bool (strict)"("DisabledEnum"=w162) -> ()  [unwired: 2 in, 2 out]
                n180 = property on="CCD3500 Preview" class="Bool (strict)"("DisabledEnum"=w162) -> ()  [unwired: 2 in, 2 out]
              }
              frame #2 {
                n181 = property on="Read CCD3500" class="Bool (strict)"("Val(Sgnl)"=TRUE ("Wert (signalisierend)")) -> ()  [unwired: 2 in, 2 out]
                n182 = property on="CCD3500V Running" class="Bool (strict)"("Blinking"=FALSE ("Blinkend")) -> ()  [unwired: 2 in, 2 out]
              }
            }
          }
          event "Read CCD3500": Value Change {
            n183 = event-data() -> ("NewVal"=w182:bool)  [unwired: 1 in, 4 out]
            n184 = local read "CCD3500V Status"() -> (w181:bool)
            n185 = And(x=w181, y=w182) -> (x .and. y?=w180:bool)
            n186 = case shown="True" w180 {
              tunnel: [u32 0 w184] -> w179
              frame False {
              }
              frame True {
                n187 = stacked-sequence {
                  seq-local: [_ w186 _ _] -> [_ _ w191 _]
                  seq-local: [w185 _ _ _] -> [_ _ _ w202]
                  tunnel: [_ _ _ w203] -> w184
                  frame #0 {
                    n188 = Tick Count (ms)() -> (millisecond timer value=w185:u32)
                  }
                  frame #1 {
                    n189 = local read "CCD3500V Connection"() -> (w190:T11)
                    n190 = call "PROPGET.VI"("CCD Prop ID"=T19."CCD Temperature Z345", "Comm Params"=w190) -> ("Output Param"=w188:dbl)  [unwired: 1 out]
                    n191 = Subtract(x=w188, y=273.15) -> (x-y=w186:dbl)
                    n192 = local write "CCD3500 Temperature"(w186) -> ()
                  }
                  frame #2 {
                    n193 = Greater?(x=w191, y=-122.0) -> (0:w192:bool)
                    n194 = case shown="True" w192 {
                      selector: w192 -> [w199 w201]
                      tunnel: [cluster{u32, u32}[] [{16713728, 16713728}, {6618880, 6618880}] ("Farben [4]") cluster{u32, u32}[] [{16713728, 16713728}] ("Farben [4]")] -> w193
                      tunnel: [w199 w201] -> w195
                      frame False {
                      }
                      frame True {
                      }
                    }
                    n195 = Number To Fractional String(number=w191, precision (6)=i16 1 ("Genauigkeit (6)")) -> (F-format string=w194:string)  [unwired: 2 in]
                    n196 = global write "Global Variables.vi" "Global CCD Temperature (C)"(w191) -> ()
                    n197 = property on="CCD3500V Status" class="Bool (strict)"("Blinking"=w195, "BoolText.Text"=w194, "Colors [4]"=w193) -> ()  [unwired: 2 in, 2 out]
                  }
                  frame #3 {
                    n198 = Tick Count (ms)() -> (millisecond timer value=w204:u32)
                    n199 = Subtract(x=w204, y=w202) -> (x-y=w203:u32)
                  }
                }
              }
            }
            "CCD Timing" <- w179
          }
          event "Drive Connect": Value Change {
            n200 = event-data() -> ("NewVal"=w205:bool)  [unwired: 1 in, 4 out]
            n201 = stacked-sequence {
              tunnel: w205 -> [_ w209 _ _]
              frame #0 {
                n202 = property on="Drive Running" class="Bool (strict)"("Blinking"=TRUE ("Blinkend")) -> ()  [unwired: 2 in, 2 out]
              }
              frame #1 {
                n203 = local read "Drive Connection"() -> (w210:T4)
                n204 = Not(x=w209) -> (.not. x?=w211:bool)
                n205 = call "ESA-C Connect.vi"("Remote=F /Local=T"=w211, "Drive Connection Settings"=w210) -> ("Success"=w212:bool)  [unwired: 2 in]
                n206 = Exclusive Or(1:w211, 2:w212) -> (0:w213:bool)
                n207 = local write "Drive Connect"(w213) -> ()
                n208 = local write "Drive Status"(w213) -> ()
                n209 = case shown="False" w213 {
                  tunnel: [T17."Disabled and Grayed Out" ("Deaktiviert") T17."Enabled" ("Deaktiviert")] -> w208
                  tunnel: ["" ("Boolescher Text.Text") w216] -> w207
                  frame False {
                  }
                  frame True {
                    n210 = property on="Drive Selector" class="Ring (strict)"() -> ("RingText.Text"=w216:string)  [unwired: 2 in, 2 out]
                  }
                }
                n211 = property on="Drive Live Controls" class="Clust (strict)"("DisabledEnum"=w208) -> ()  [unwired: 2 in, 2 out]
                n212 = property on="Drive Status" class="Bool (strict)"("BoolText.Text"=w207) -> ()  [unwired: 2 in, 2 out]
                n213 = property on="Drive GoTo" class="Bool (strict)"("DisabledEnum"=w208) -> ()  [unwired: 2 in, 2 out]
              }
              frame #2 {
                # "prepare mirroring values to target controls"
                n214 = local write "Copy Drive Target"(TRUE ("Copy Drive Target")) -> ()
              }
              frame #3 {
                n215 = property on="Drive Running" class="Bool (strict)"("Blinking"=FALSE ("Blinkend")) -> ()  [unwired: 2 in, 2 out]
                n216 = property on="Read Drive" class="Bool (strict)"("Val(Sgnl)"=TRUE ("Wert (signalisierend)")) -> ()  [unwired: 2 in, 2 out]
              }
            }
          }
          event "Read Drive": Value Change {
            n217 = event-data() -> ("NewVal"=w224:bool)  [unwired: 1 in, 4 out]
            n218 = local read "Drive Status"() -> (w223:bool)
            n219 = And(x=w223, y=w224) -> (x .and. y?=w222:bool)
            n220 = case shown="True" w222 {
              tunnel: [u32 0 w226] -> w221
              frame False {
              }
              frame True {
                n221 = stacked-sequence {
                  seq-local: [w227 _ _ _] -> [_ _ _ w233]
                  tunnel: [_ _ _ w232] -> w226
                  frame #0 {
                    n222 = Tick Count (ms)() -> (millisecond timer value=w227:u32)
                  }
                  frame #1 {
                    n223 = local read "Drive Connection"() -> (w229:T4)
                    n224 = call "ESA-C Get Values.vi"("Drive Connection Settings"=w229) -> ("Drive Current Values"=w228:T3)
                    n225 = local write "Drive Live Current Values"(w228) -> ()
                    n226 = local write "Drive Current Values"(w228) -> ()
                    n227 = global write "Global Variables.vi" "Global Drive Position"(w228) -> ()
                  }
                  frame #2 {
                    n228 = local read "Copy Drive Target"() -> (w230:bool)
                    n229 = case shown="True" w230 {
                      frame False {
                      }
                      frame True {
                        n230 = property on="Copy Drive Target" class="Bool (strict)"("Val(Sgnl)"=TRUE ("Value (Signaling)")) -> ()  [unwired: 2 in, 2 out]
                      }
                    }
                  }
                  frame #3 {
                    n231 = Tick Count (ms)() -> (millisecond timer value=w234:u32)
                    n232 = Subtract(x=w234, y=w233) -> (x-y=w232:u32)
                  }
                }
              }
            }
            "Drive Timing" <- w221
          }
          event "Copy Drive Target": Value Change {
            # "this event is triggered after drive readout\nit should usually not be triggered directly by signaling"
            n233 = event-data() -> ("NewVal"=w235:bool)  [unwired: 1 in, 4 out]
            n234 = case shown="True" w235 {
              frame False {
              }
              frame True {
                n235 = stacked-sequence {
                  frame #0 {
                    n236 = local read "Drive Current Values"() -> (w237:T3)
                    n237 = Unbundle By Name(w237) -> ("Position"=w236:T21)
                    n238 = local write "Drive New Positions"(w236) -> ()
                  }
                  frame #1 {
                    n239 = local write "Copy Drive Target"(FALSE ("Copy Drive Target")) -> ()
                  }
                }
              }
            }
          }
          event "Video Show": Value Change {
            n240 = event-data() -> ("NewVal"=w239:bool)  [unwired: 1 in, 4 out]
            n241 = case shown="True" w239 {
              frame False {
              }
              frame True {
                w240 = "true" ("Control Name")
                n242 = vi-ref "Video Toolset v10.0.0.vi"() -> (w256:refnum<vi>)
                n243 = invoke class="VI" method="Ctrl Val.Set"(reference=w256, "Control Name"="AutorunText", "Value"=w240) -> (reference out=w245:refnum<vi>, error out=w244:errorcluster)  [unwired: 2 in, 3 out]
                n244 = invoke class="VI" method="Ctrl Val.Set"(reference=w245, error in=w244, "Control Name"="AutocloseText", "Value"=w240) -> (reference out=w241:refnum<vi>, error out=w242:errorcluster)  [unwired: 1 in, 3 out]
                n245 = local read "Camera Name"() -> (w248:string)
                n246 = local read "Snapshot Folder"() -> (w247:path)
                n247 = invoke class="VI" method="Ctrl Val.Set"(reference=w241, error in=w242, "Control Name"="Source Name", "Value"=w248) -> (reference out=w253:refnum<vi>, error out=w252:errorcluster)  [unwired: 1 in, 3 out]
                n248 = invoke class="VI" method="Ctrl Val.Set"(reference=w253, error in=w252, "Control Name"="Capture Folder", "Value"=w247) -> (reference out=w254:refnum<vi>, error out=w255:errorcluster)  [unwired: 1 in, 3 out]
                n249 = invoke on="Invoke Node" class="VI" method="FP.Open"(reference=w254, error in=w255, "Activate"=TRUE ("Activate?")) -> (reference out=w258:refnum<vi>, error out=w257:errorcluster)  [unwired: 2 in, 3 out]
                n250 = local write "Video Show"(FALSE ("Video Show")) -> ()
                n251 = invoke on="Invoke Node" class="VI" method="Run VI"(reference=w258, error in=w257, "Wait until done"=FALSE ("Wait Until Done"), "Auto Dispose Ref"=TRUE ("Auto Dispose Reference")) -> ()  [unwired: 1 in, 5 out]
              }
            }
          }
          event "ITC503 Configure": Value Change {
            n252 = event-data() -> ("NewVal"=w262:bool)  [unwired: 1 in, 4 out]
            n253 = stacked-sequence {
              tunnel: w262 -> [_ w264 _]
              frame #0 {
                n254 = property on="ITC503s Running" class="Bool (strict)"("Blinking"=TRUE ("Blinkend")) -> ()  [unwired: 2 in, 2 out]
              }
              frame #1 {
                n255 = local read "ITC503 Status"() -> (w266:bool)
                n256 = And(x=w266, y=w264) -> (x .and. y?=w265:bool)
                n257 = case shown="True" w265 {
                  frame False {
                  }
                  frame True {
                    n258 = local read "ITC503 Settings"() -> (w267:T2)
                    n259 = local read "ITC Setup"() -> (w268:T12)
                    n260 = call "ITC503 Set Values.vi"("Set Channel"=i16 1, "ITC503 Settings"=w267, "ITC Setup"=w268) -> ()  [unwired: 2 in]
                  }
                }
              }
              frame #2 {
                w271 = FALSE ("Blinkend")
                n261 = local write "ITC503 Configure"(w271) -> ()
                n262 = property on="ITC503s Running" class="Bool (strict)"("Blinking"=w271) -> ()  [unwired: 2 in, 2 out]
                n263 = property on="Read ITC" class="Bool (strict)"("Val(Sgnl)"=TRUE ("Wert (signalisierend)")) -> ()  [unwired: 2 in, 2 out]
              }
            }
          }
          event "iHR550 Configure": Value Change {
            n264 = event-data() -> ("NewVal"=w272:bool)  [unwired: 1 in, 4 out]
            n265 = stacked-sequence {
              tunnel: w272 -> [_ w274 _]
              frame #0 {
                n266 = property on="iHR550 Running" class="Bool (strict)"("Blinking"=TRUE ("Blinkend")) -> ()  [unwired: 2 in, 2 out]
              }
              frame #1 {
                n267 = local read "iHR550 Status"() -> (w276:bool)
                n268 = local read "iHR550 RefNum"() -> (w277:refnum<k7>)
                n269 = And(x=w276, y=w274) -> (x .and. y?=w275:bool)
                n270 = case shown="True" w275 {
                  tunnel: w277 -> [_ w278]
                  frame False {
                  }
                  frame True {
                    n271 = stacked-sequence {
                      seq-local: [_ w283 _] -> [_ _ w286]
                      tunnel: w278 -> [w279 w284 _]
                      frame #0 {
                        w282 = u16 2 items=["Front"=2, "Side"=3] ("Entrance Mirror")
                        n272 = local read "iHR Settings"() -> (w280:T7)
                        n273 = call "iHR550 Set Values.vi"("Refnum out"=w279, "Entrance Mirror"=w282, "Target\nSide Entrance"=0.0 ("Target\nSide Entrance"), "iHR Settings"=w280) -> ()  [unwired: 11 in, 1 out]
                      }
                      frame #1 {
                        n274 = call "iHR550 Read Values.vi"("JYMONOLib.IJYMonoReqd"=w284) -> ("iHR Current Values"=w283:T8)  [unwired: 1 in]
                        n275 = local write "iHR Current Values"(w283) -> ()
                      }
                      frame #2 {
                        n276 = call "iHR550 Convert Axis.vi"("iHR Current Values"=w286) -> ("Wavelengths (nm)"=w285:dbl[])
                        n277 = local write "Wavelengths (nm)"(w285) -> ()
                        n278 = global write "Global Variables.vi" "Global Wavelengths (nm)"(w285) -> ()
                      }
                    }
                  }
                }
              }
              frame #2 {
                w288 = FALSE ("Blinkend")
                n279 = property on="Read iHR550" class="Bool (strict)"("Val(Sgnl)"=TRUE ("Wert (signalisierend)")) -> ()  [unwired: 2 in, 2 out]
                n280 = local write "iHR550 Configure"(w288) -> ()
                n281 = property on="iHR550 Running" class="Bool (strict)"("Blinking"=w288) -> ()  [unwired: 2 in, 2 out]
              }
            }
          }
          event "CCD3500 Preview": Value Change {
            n282 = event-data() -> ("NewVal"=w289:bool)  [unwired: 1 in, 4 out]
            n283 = case shown="True" w289 {
              frame False {
              }
              frame True {
                n284 = property on="CCD3500 Acquire" class="Bool (strict)"("Val(Sgnl)"=TRUE ("Wert (signalisierend)")) -> ()  [unwired: 2 in, 2 out]
              }
            }
          }
          event "CCD3500 Acquire": Value Change {
            n285 = event-data() -> ("NewVal"=w291:bool)  [unwired: 1 in, 4 out]
            n286 = stacked-sequence {
              tunnel: w291 -> [w292 _]
              frame #0 {
                n287 = case shown="True" w292 {
                  frame False {
                  }
                  frame True {
                    n288 = local read "CCD3500V Connection"() -> (w293:T11)
                    n289 = local read "Spectra Settings"() -> (w294:T6)
                    n290 = stacked-sequence {
                      tunnel: w294 -> [w297 w309 _]
                      tunnel: w293 -> [w296 w305 _]
                      frame #0 {
                        # "prepare acquisition if settings changed"
                        n291 = Unbundle By Name(w297) -> ("Integration Time"=w295:dbl)
                        n292 = local read "Int. Time Temp"() -> (w298:dbl)
                        n293 = Equal?(x=w295, y=w298) -> (x = y?=w299:bool)
                        n294 = case shown="False" w299 {
                          tunnel: w298 -> [_ _]
                          tunnel: w297 -> [w302 _]
                          tunnel: w296 -> [w301 _]
                          tunnel: w295 -> [w300 _]
                          frame False {
                            n295 = call "CCD3000 Prepare Acquisition.vi"("Mapping Spectra Settings"=w302, "Comm Params"=w301) -> ()  [unwired: 4 in]
                            n296 = local write "Int. Time Temp"(w300) -> ()
                          }
                          frame True {
                          }
                        }
                      }
                      frame #1 {
                        n297 = local read "CCD3500 Preview"() -> (w308:bool)
                        n298 = Unbundle By Name(w309) -> ("Repetitions"=w306:u16)
                        n299 = Select(t=i8 1, s=w308, f=w306) -> (s? t:f=w304:u16)
                        n300 = for {
                          N: w304 -> [w319]
                          tunnel: w305 -> [w331]
                          shift-right: [w326] -> _
                          shift-left: u16[][] [] -> [w329]
                          i -> [w320]
                          stop <- w325 continue-if-true
                          n301 = control-ref of="CCD3500 Acquire"() -> (w324:refnum<vi>)
                          n302 = control-ref of="CCD3500V Running"() -> (w323:refnum<vi>)
                          n303 = call "CCD3000 Spectral Acquisition.vi"("Acquire"=w324, "Running"=w323, "Comm Params"=w331) -> ("Raw-Spectrum"=w330:u16[])  [unwired: 6 in, 2 out]
                          n304 = Number To Decimal String(number=w319) -> (decimal integer string=w318:string)  [unwired: 1 in]
                          n305 = Build Array (concatenate)(w330, w329) -> (w326:u16[][])
                          n306 = Increment(x=w320) -> (x+1=w316:i32)
                          n307 = Number To Decimal String(number=w316) -> (decimal integer string=w317:string)  [unwired: 1 in]
                          n308 = local read "Wavelengths (nm)"() -> (w328:dbl[])
                          n309 = local read "Spectrum Noise"() -> (w315:i64)
                          n310 = Concatenate Strings(w317, "/" ("string"), w318) -> (w322:string)
                          n311 = call "CCD3000 Average Spectra.vi"("Repetitions"=w316, "Raw Spectra"=w326) -> ("Raw Spectrum"=w327:dbl[])
                          n312 = local read "Wavelength Switch"() -> (w314:bool)
                          n313 = local write "CCD3000 Current Rep."(w322) -> ()
                          n314 = call "CCD3000 Pixel to Wavelength v10.1.0.vi"("Wavelengths (nm)"=w328, "Raw Spectrum"=w327) -> ("Spectrum-Array"=w310:dbl[][])  [unwired: 1 out]
                          n315 = call "CCD3000 Noise Subtraction v10.4.0.vi"("Spectrum Noise"=w315, "Spectrum-Array In"=w310) -> ("Spectrum-Array Out"=w313:dbl[][], "Spectrum-Cluster"=w311:T22)
                          n316 = local write "Spectrum Raw"(w310) -> ()
                          n317 = case shown="False" w314 {
                            tunnel: w313 -> [_ w334]
                            tunnel: [w332 w333] -> w312
                            tunnel: w311 -> [w332 _]
                            frame False {
                            }
                            frame True {
                              n318 = call "CCD3000 Jacobian Transformation v10.4.0.vi"("Spectrum-Array In"=w334) -> ("Spectrum-Cluster"=w333:T22)  [unwired: 1 in, 1 out]
                            }
                          }
                          n319 = local read "CCD3500 Acquire"() -> (w325:bool)
                          n320 = local write "Spectrum"(w312) -> ()
                        }
                      }
                      frame #2 {
                        n321 = local read "Spectrum Autosave"() -> (w335:bool)
                        n322 = case shown="True" w335 {
                          frame False {
                          }
                          frame True {
                            n323 = property on="Spectrum Save" class="Bool (strict)"("Val(Sgnl)"=TRUE ("Value (Signaling)")) -> ()  [unwired: 2 in, 2 out]
                          }
                        }
                      }
                    }
                  }
                }
              }
              frame #1 {
                n324 = local write "CCD3500 Acquire"(FALSE ("Blinkend")) -> ()
                n325 = local write "CCD3000 Current Rep."("0/0" ("CCD3000 Current Rep.")) -> ()
              }
            }
          }
          event "Wavelength Switch": Value Change {
            n326 = event-data() -> ("NewVal"=w339:bool)  [unwired: 1 in, 4 out]
            n327 = case shown="True" w339 {
              frame False {
                n328 = local read "Spectrum Noise"() -> (w340:i64)
                n329 = local read "Spectrum Raw"() -> (w341:dbl[][])
                n330 = property on="Spectrum" class="XYGraph (strict)"("XScale.NameLbl.Text"="Wavelenght (nm)" ("X Scale.Name Label.Text")) -> ()  [unwired: 2 in, 2 out]
                n331 = call "CCD3000 Noise Subtraction v10.4.0.vi"("Spectrum Noise"=w340, "Spectrum-Array In"=w341) -> ("Spectrum-Cluster"=w342:T22)  [unwired: 1 out]
                n332 = local write "Spectrum"(w342) -> ()
              }
              frame True {
                # "Jacobian Transformation requires noise subtraction"
                n333 = local read "Spectrum Noise"() -> (w345:i64)
                n334 = Greater Than 0?(x=w345) -> (x > 0?=w344:bool)
                n335 = case shown="False" w344 {
                  frame False {
                    n336 = call "Display Message to User"() -> ()  [unwired: 10 in, 2 out]
                    n337 = local write "Wavelength Switch"(FALSE ("Wavelength Switch")) -> ()
                  }
                  frame True {
                    n338 = local read "Spectrum Noise"() -> (w347:i64)
                    n339 = local read "Spectrum Raw"() -> (w348:dbl[][])
                    n340 = property on="Spectrum" class="XYGraph (strict)"("XScale.NameLbl.Text"="Energy (eV)" ("X Scale.Name Label.Text")) -> ()  [unwired: 2 in, 2 out]
                    n341 = call "CCD3000 Noise Subtraction v10.4.0.vi"("Spectrum Noise"=w347, "Spectrum-Array In"=w348) -> ("Spectrum-Array Out"=w349:dbl[][])  [unwired: 1 out]
                    n342 = call "CCD3000 Jacobian Transformation v10.4.0.vi"("Spectrum-Array In"=w349) -> ("Spectrum-Cluster"=w350:T22)  [unwired: 1 in, 1 out]
                    n343 = local write "Spectrum"(w350) -> ()
                  }
                }
              }
            }
          }
          event "Spectrum Noise": Value Change {
            n344 = event-data() -> ("NewVal"=w353:i64)  [unwired: 1 in, 4 out]
            n345 = Greater Than 0?(x=w353) -> (x > 0?=w352:bool)
            n346 = stacked-sequence {
              tunnel: w352 -> [w354 _]
              frame #0 {
                n347 = case shown="True" w354 {
                  frame False {
                    # "Disable Jacobian Transformation"
                    n348 = local write "Wavelength Switch"(FALSE ("Wavelength Switch")) -> ()
                  }
                  frame True {
                  }
                }
              }
              frame #1 {
                n349 = local read "Wavelength Switch"() -> (w356:bool)
                n350 = local read "Spectrum Noise"() -> (w361:i64)
                n351 = local read "Spectrum Raw"() -> (w360:dbl[][])
                n352 = call "CCD3000 Noise Subtraction v10.4.0.vi"("Spectrum Noise"=w361, "Spectrum-Array In"=w360) -> ("Spectrum-Array Out"=w359:dbl[][], "Spectrum-Cluster"=w357:T22)
                n353 = case shown="False" w356 {
                  tunnel: w359 -> [_ w364]
                  tunnel: [w362 w363] -> w358
                  tunnel: w357 -> [w362 _]
                  frame False {
                  }
                  frame True {
                    n354 = call "CCD3000 Jacobian Transformation v10.4.0.vi"("Spectrum-Array In"=w364) -> ("Spectrum-Cluster"=w363:T22)  [unwired: 1 in, 1 out]
                  }
                }
                n355 = local write "Spectrum"(w358) -> ()
              }
            }
          }
          event "CCD3500 Shutter": Value Change {
            n356 = event-data() -> ("NewVal"=w365:bool)  [unwired: 1 in, 4 out]
            n357 = local read "CCD3500V Status"() -> (w366:bool)
            n358 = case shown="True" w366 {
              tunnel: w365 -> [_ w369]
              frame False {
              }
              frame True {
                n359 = local read "CCD3500V Connection"() -> (w368:T11)
                n360 = call "CCD Shutter.vi"("Shutter"=w369, "Comm Params"=w368) -> ("Error"=w367:bool)
                n361 = case shown="True" w367 {
                  tunnel: w369 -> [_ w370]
                  frame False {
                  }
                  frame True {
                    n362 = Not(x=w370) -> (.not. x?=w371:bool)
                    n363 = local write "CCD3500 Shutter"(w371) -> ()
                  }
                }
              }
            }
          }
          event "Drive GoTo": Value Change {
            n364 = event-data() -> ("NewVal"=w372:bool)  [unwired: 1 in, 4 out]
            n365 = stacked-sequence {
              tunnel: w372 -> [_ w374 _]
              frame #0 {
                n366 = property on="Drive Running" class="Bool (strict)"("Blinking"=TRUE ("Blinkend")) -> ()  [unwired: 2 in, 2 out]
              }
              frame #1 {
                n367 = local read "Drive Status"() -> (w376:bool)
                n368 = And(x=w376, y=w374) -> (x .and. y?=w375:bool)
                n369 = case shown="True" w375 {
                  frame False {
                  }
                  frame True {
                    n370 = local read "Drive New Positions"() -> (w377:T5)
                    n371 = local read "Drive Connection"() -> (w378:T4)
                    n372 = control-ref of="Drive Running"() -> (w379:refnum<vi>)
                    n373 = call "ESA-C Move Absolute.vi"("Running"=w379, "Drive New Abs. Positions"=w377, "Drive Connection Settings"=w378) -> ()  [unwired: 2 in]
                  }
                }
              }
              frame #2 {
                w381 = FALSE ("Blinkend")
                n374 = local write "Drive GoTo"(w381) -> ()
                n375 = property on="Drive Running" class="Bool (strict)"("Blinking"=w381) -> ()  [unwired: 2 in, 2 out]
                n376 = property on="Read Drive" class="Bool (strict)"("Val(Sgnl)"=TRUE ("Wert (signalisierend)")) -> ()  [unwired: 2 in, 2 out]
              }
            }
          }
          event Value Change {
            n377 = event-data() -> ("NewVal"=w383:bool)  [unwired: 1 in, 4 out]
            n378 = local read "Drive Status"() -> (w384:bool)
            n379 = And(x=w384, y=w383) -> (x .and. y?=w382:bool)
            n380 = case shown="True" w382 {
              frame False {
              }
              frame True {
                n381 = stacked-sequence {
                  seq-local: [w385 _ _] -> [_ _ _]
                  frame #0 {
                    # "Move and Read"
                    n382 = flat-sequence {
                      tunnel: [w392] -> w388
                      tunnel: [w389] -> w387
                      tunnel: w388 -> [w394]
                      tunnel: w387 -> [w395]
                      tunnel: [w393] -> w386
                      tunnel: w386 -> [w400]
                      tunnel: [w400] -> w385
                      frame #0 {
                        n383 = local read "Drive Live Controls"() -> (w389:T9)
                        n384 = local read "Drive Connection"() -> (w390:T4)
                        n385 = control-ref of="Drive Running"() -> (w391:refnum<vi>)
                        n386 = call "ESA-C Live Control v10.4.0.vi"("Running"=w391, "Drive Live Controls"=w389, "Drive Connection Settings"=w390) -> ("Reset Switches"=w392:bool)  [unwired: 1 in]
                      }
                      frame #1 {
                        n387 = case shown="True" w394 {
                          tunnel: w395 -> [w396 w399]
                          tunnel: [w396 w398] -> w393
                          frame False {
                          }
                          frame True {
                            w397 = FALSE ("Move Out")
                            n388 = Bundle By Name(cluster=w399, "Move Home"=w397, "Move Down"=w397, "Move Up"=w397, "Move Left"=w397, "Move Right"=w397, "Move Out"=w397, "Move In"=w397) -> (w398:T9)
                          }
                        }
                      }
                      frame #2 {
                        n389 = local write "Drive Live Controls"(w400) -> ()
                      }
                    }
                  }
                  frame #1 {
                    n390 = local write "Copy Drive Target"(TRUE ("Copy Drive Target")) -> ()
                  }
                  frame #2 {
                    n391 = property on="Read Drive" class="Bool (strict)"("Val(Sgnl)"=TRUE ("Wert (signalisierend)")) -> ()  [unwired: 2 in, 2 out]
                  }
                }
              }
            }
          }
          event "Spectrum Save": Value Change {
            n392 = event-data() -> ("NewVal"=w403:bool)  [unwired: 1 in, 4 out]
            n393 = stacked-sequence {
              tunnel: w403 -> [w404 _]
              frame #0 {
                n394 = case shown="True" w404 {
                  frame False {
                  }
                  frame True {
                    n395 = local read "CCD3500 Temperature"() -> (w410:dbl)
                    n396 = local read "ITC503 Current Values"() -> (w411:T1)
                    n397 = local read "Drive Current Values"() -> (w412:T3)
                    n398 = local read "iHR Current Values"() -> (w414:T8)
                    n399 = local read "Spectra Settings"() -> (w413:T6)
                    n400 = local read "Spectrum Raw"() -> (w405:dbl[][])
                    n401 = call "Export_spectrumFileName.vi"("ITC503 Current Values"=w411, "iHR Current Values"=w414, "Spectra Settings"=w413, "Drive Current Values"=w412, "CCD3500 Temperature"=w410) -> ("Filename"=w409:string)
                    n402 = local read "Spectrum Autosave"() -> (w407:bool)
                    n403 = local read "Auto Folder"() -> (w406:path)
                    n404 = call "Export_2DtoTxt v10.2.0.vi"("Auto Folder"=w406, "Auto?"=w407, "Data (2D)"=w405, "Export Type"="Spectrum", "Filename"=w409) -> ()  [unwired: 1 in]
                  }
                }
              }
              frame #1 {
                n405 = local write "Spectrum Save"(FALSE ("Spectrum Save")) -> ()
              }
            }
          }
          event "Spectrum Load": Value Change {
            n406 = event-data() -> ("NewVal"=w416:bool)  [unwired: 1 in, 4 out]
            n407 = case shown="True" w416 {
              frame False {
              }
              frame True {
                n408 = stacked-sequence {
                  seq-local: [w417 _ _] -> [_ w420 _]
                  frame #0 {
                    n409 = call "Load Spectrum.vi"() -> ("Intensity"=w417:dbl[], "Wavelength"=w419:dbl[])  [unwired: 3 in, 1 out]
                    n410 = Build Array(w419, w417) -> (w418:dbl[][])
                    n411 = local write "Spectrum Raw"(w418) -> ()
                  }
                  frame #1 {
                    n412 = call <vilib>:"Median.vi"("X"=w420) -> ("median"=w422:dbl)  [unwired: 1 out]
                    n413 = To Long Integer(number=w422) -> (32bit integer=w421:i32)
                    n414 = property on="Spectrum Noise" class="DigNum (strict)"("Val(Sgnl)"=w421) -> ()  [unwired: 2 in, 2 out]
                  }
                  frame #2 {
                    n415 = local write "Spectrum Load"(FALSE ("Spectrum Load")) -> ()
                  }
                }
              }
            }
          }
          event "Spectrum Autosave": Value Change {
            n416 = event-data() -> ("NewVal"=w425:bool)  [unwired: 1 in, 4 out]
            n417 = case shown="True" w425 {
              tunnel: [path "" w431] -> w424
              frame False {
              }
              frame True {
                n418 = call "File Dialog"("prompt"="Choose Save Folder") -> ("selected path"=w433:path, "cancelled"=w427:bool, "error out"=w429:errorcluster)  [unwired: 11 in, 1 out]
                n419 = call <vilib>:"Simple Error Handler.vi"("error in (no error)"=w429) -> ("error?"=w428:bool)  [unwired: 4 in, 4 out]
                n420 = Or(x=w427, y=w428) -> (x .or. y?=w430:bool)
                n421 = case shown="True" w430 {
                  tunnel: w433 -> [w434 _]
                  tunnel: [w434 path ""] -> w431
                  frame False {
                  }
                  frame True {
                    n422 = local write "Spectrum Autosave"(FALSE ("Spectrum Autosave")) -> ()
                  }
                }
              }
            }
            n423 = local write "Auto Folder"(w424) -> ()
          }
          event "Spectrum Maximize": Value Change {
            # "Currently disabled by hiding control!"
            n424 = event-data() -> ("NewVal"=w437:bool)  [unwired: 1 in, 4 out]
            n425 = case shown="True" w437 {
              frame False {
                n426 = local read "Spectrum Properties"() -> (w440:cluster{"Position":T10, "Plot Area Size":T10})
                n427 = Unbundle(w440) -> ("Position"=w439:T10, "Plot Area Size"=w438:T10)
                n428 = stacked-sequence {
                  tunnel: w439 -> [_ w442]
                  tunnel: w438 -> [w441 _]
                  frame #0 {
                    n429 = property on="Spectrum" class="XYGraph (strict)"("Plot Area Size"=w441) -> ()  [unwired: 2 in, 2 out]
                  }
                  frame #1 {
                    n430 = property on="Spectrum" class="XYGraph (strict)"("Position"=w442) -> ()  [unwired: 2 in, 2 out]
                  }
                }
              }
              frame True {
                n431 = property on="Spectrum" class="XYGraph (strict)"() -> ("Bounds"=w463:T10, "Plot Area Size"=w462:T10, "Position"=w460:T23)  [unwired: 2 in, 2 out]
                n432 = Bundle("Position"=w460, "Plot Area Size"=w462) -> (w461:cluster{"Position":T23, "Plot Area Size":T10})  [unwired: 1 in]
                n433 = Unbundle By Name(w463) -> ("Width"=w467:u32, "Height"=w468:u32)
                n434 = Unbundle By Name(w462) -> ("Width"=w470:u32, "Height"=w469:u32)
                n435 = property on="Register" class="TabCtl (strict)"() -> ("Bounds"=w466:T10, "Position"=w455:T23, "Width"=w446:u32, "Height"=w445:u32)  [unwired: 2 in, 2 out]
                n436 = local write "Spectrum Properties"(w461) -> ()
                n437 = Subtract(x=w467, y=w470) -> (x-y=w459:u32)
                n438 = Subtract(x=w468, y=w469) -> (x-y=w456:u32)
                n439 = Add(x=w459, y=u32 25) -> (x+y=w458:u32)
                n440 = Add(x=w456, y=u32 70) -> (x+y=w457:u32)
                n441 = Subtract(x=w446, y=w458) -> (x-y=w465:u32)
                n442 = Subtract(x=w445, y=w457) -> (x-y=w464:u32)
                n443 = Bundle By Name(cluster=w466, "Width"=w465, "Height"=w464) -> (w443:T10)
                n444 = Unbundle By Name(w455) -> ("Left"=w454:i32, "Top"=w451:i32)
                n445 = Add(x=w454, y=20) -> (x+y=w453:i32)
                n446 = Add(x=w451, y=50) -> (x+y=w452:i32)
                n447 = Bundle By Name(cluster=w455, "Left"=w453, "Top"=w452) -> (w444:T23)
                n448 = stacked-sequence {
                  tunnel: w444 -> [w471 _]
                  tunnel: w443 -> [_ w472]
                  frame #0 {
                    n449 = property on="Spectrum" class="XYGraph (strict)"("Position"=w471) -> ()  [unwired: 2 in, 2 out]
                  }
                  frame #1 {
                    n450 = property on="Spectrum" class="XYGraph (strict)"("Plot Area Size"=w472) -> ()  [unwired: 2 in, 2 out]
                  }
                }
              }
            }
          }
          event "Mapping Start": Value Change {
            n451 = event-data() -> ("NewVal"=w473:bool)  [unwired: 1 in, 4 out]
            n452 = case shown="True" w473 {
              frame False {
              }
              frame True {
                n453 = local read "CCD3500V Status"() -> (w500:bool)
                n454 = local read "CCD3500V Connection"() -> (w509:T11)
                n455 = local read "CCD3500 Temperature"() -> (w511:dbl)
                n456 = local read "ITC503 Current Values"() -> (w506:T1)
                n457 = local read "Drive Current Values"() -> (w504:T3)
                n458 = vi-ref "Mapping v10.4.0.vi"() -> (w491:refnum<vi>)
                n459 = local read "iHR Current Values"() -> (w505:T8)
                n460 = local read "Wavelengths (nm)"() -> (w507:dbl[])
                n461 = local read "Drive Status"() -> (w502:bool)
                n462 = local read "Drive Connection"() -> (w508:T4)
                n463 = local read "Spectra Settings"() -> (w510:T6)
                n464 = local read "CCD3500V Status"() -> (w484:bool)
                n465 = Not(x=w502) -> (.not. x?=w501:bool)
                n466 = Not(x=w500) -> (.not. x?=w499:bool)
                n467 = Not(x=w484) -> (.not. x?=w483:bool)
                n468 = Bundle By Name(cluster=T20 {"CCD3000 Connection"={"Comm Interface"=1, "BUS"=0, "Address"=5, "Com Port"=1}, "Drive Connection Settings"={"Objective GPIB-Port"=4, "Stage GPIB-Port"=4, "Drive Selector"=0, "Drive Velocity (V/s)"=5.0}, "ITC503 Current Values"={"ITC503 Heater"=0.0, "ITC503 Temperature"=0.0, "ITC503 P"=0.0, "ITC503 I"=0.0, "ITC503 D"=0.0, "ITC503 Setpoint"=0.0, "ITC503 Gradient"=0.0, "ITC503 Heater Auto"=FALSE, "ITC503 PID Auto"=FALSE}, "Wavelengths (nm)"=[], "Drive Current Values"={"Voltages"={"Drive X Voltage"=0.0, "Drive Y Voltage"=0.0, "Drive Z Voltage"=0.0}, "Position"={"Drive X Position"=0.0, "Drive Y Position"=0.0, "Drive Z Position"=0.0}}, "iHR Current Values"={"iHR 550 Front Entrance"=0.0, "iHR550 Side Exit"=0.0, "iHR550 Wavelength"=897.9988, "iHR550 Exit Mirror"=2, "iHR550 Grating"="1", "Grating Index"=1}, "Spectra Settings"={"Integration Time"=1.0, "Repetitions"=1, "Mapping Spectra"=TRUE}, "CCD3500 Temperature"=0.0, "Simulate Drive 2"=FALSE, "Simulate Spectra 2"=FALSE} ("Input Parameters"), "CCD3000 Connection"=w509, "Drive Connection Settings"=w508, "ITC503 Current Values"=w506, "Wavelengths (nm)"=w507, "Drive Current Values"=w504, "iHR Current Values"=w505, "Spectra Settings"=w510, "CCD3500 Temperature"=w511, "Simulate Drive 2"=w501, "Simulate Spectra 2"=w499) -> (w492:T20)
                n469 = invoke class="VI" method="Ctrl Val.Set"(reference=w491, "Control Name"="Simulate Spectra", "Value"=w483) -> (reference out=w490:refnum<vi>, error out=w485:errorcluster)  [unwired: 2 in, 3 out]
                n470 = local read "Drive Status"() -> (w482:bool)
                n471 = Not(x=w482) -> (.not. x?=w481:bool)
                n472 = invoke class="VI" method="Ctrl Val.Set"(reference=w490, error in=w485, "Control Name"="Simulate Drive", "Value"=w481) -> (reference out=w489:refnum<vi>, error out=w486:errorcluster)  [unwired: 1 in, 3 out]
                n473 = invoke class="VI" method="Ctrl Val.Set"(reference=w489, error in=w486, "Control Name"="Input Parameters", "Value"=w492) -> (reference out=w479:refnum<vi>, error out=w476:errorcluster)  [unwired: 1 in, 3 out]
                n474 = property on="Measurement Running" class="Bool (strict)"("Blinking"=TRUE ("Blinkend")) -> ()  [unwired: 2 in, 2 out]
                n475 = invoke class="VI" method="Ctrl Val.Set"(reference=w479, error in=w476, "Control Name"="AutoClose", "Value"=TRUE ("Blinkend")) -> (reference out=w478:refnum<vi>, error out=w477:errorcluster)  [unwired: 1 in, 3 out]
                n476 = invoke on="Invoke Node" class="VI" method="FP.Open"(reference=w478, error in=w477, "Activate"=TRUE ("Activate?")) -> (reference out=w494:refnum<vi>, error out=w493:errorcluster)  [unwired: 2 in, 3 out]
                n477 = invoke on="Invoke Node" class="VI" method="Run VI"(reference=w494, error in=w493, "Wait until done"=FALSE ("Wait Until Done"), "Auto Dispose Ref"=TRUE ("Auto Dispose Reference")) -> ()  [unwired: 1 in, 5 out]
              }
            }
          }
        }
      }
    }
    frame #3 {
      # "Close Connections"
      n478 = control-ref of="Dieses VI"() -> (w512:refnum<vi>)
      n479 = invoke class="VI" method="Default Vals.Reinit All"(reference=w512) -> ()  [unwired: 2 in, 3 out]
    }
  }
